vi "Find Path.vi"(7 "Map Colour Coding":T1={"Empty"=16448250, "Walls"=0, "Path"=3381759, "Waypoint"=16860, "Goal"=16711680}, 8 "Diagonals":bool, 9 "Ball Data":T3, 10 "Goal":cluster{"X":sgl, "Y":sgl}, 11 "Maze Walls":T2) -> (1 "Waypoints":i32[][](array[numeric]), 2 "Full Path":i32[][](array[numeric]), 3 "Image Out":T2)   [LabVIEW 2012]
uses:
  <vilib>/vision/Image Controls.llb/IMAQ Image.ctl
  <vilib>/robotics/Navigation/shared/WorldMap/OccupancyGridWorldMap/NI_Robotics_OccupancyGridWorldMap.lvclass
  <vilib>/robotics/Navigation/NI_Robotics_Navigation .lvlib
  <vilib>/vision/NI_Vision_Development_Module.lvlib
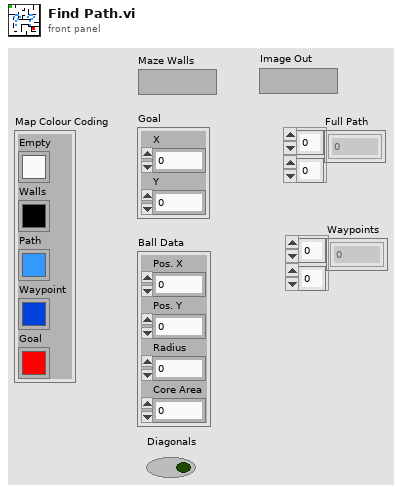
[diagram p1: front panel]
types:
  T1 = cluster{"Empty":u32, "Walls":u32, "Path":u32, "Waypoint":u32, "Goal":u32}
  T2 = typedef "IMAQ Image.ctl" = refnum<image>
  T3 = cluster{"Pos. X":i32, "Pos. Y":i32, "Radius":i32, "Core Area":i32}
  T4 = typedef "Image Type" = u32
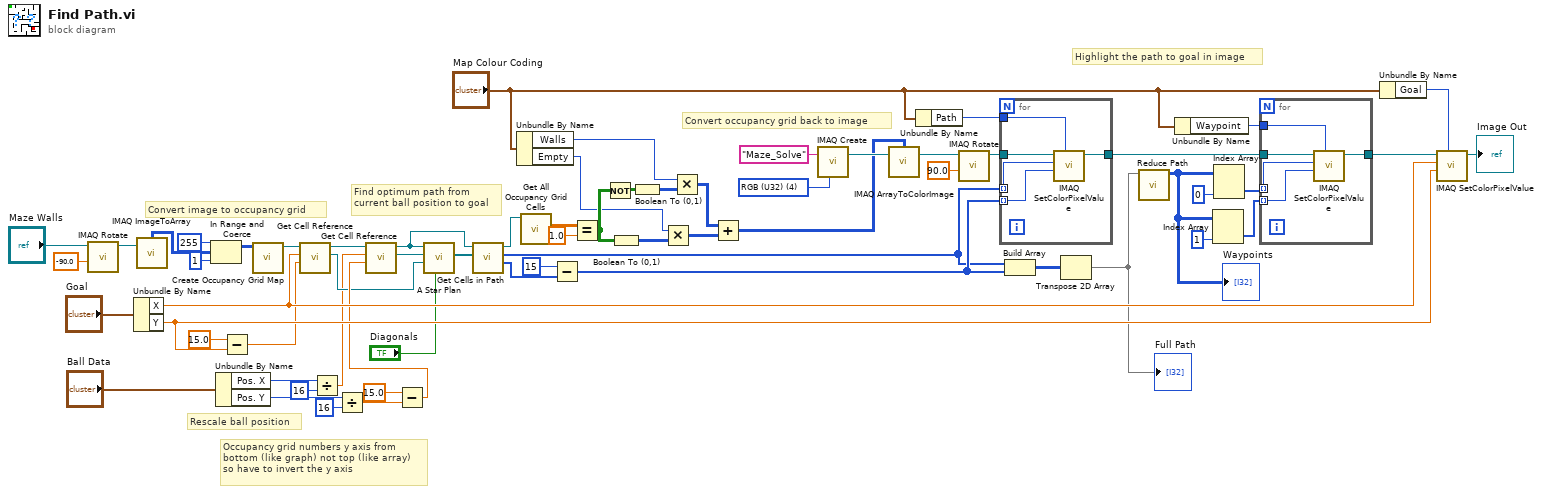
[diagram p0: block diagram]
diagram:
  w53 = T4 4 items=["Grayscale (U8)", "Grayscale (I16)", "Grayscale (SGL)", "Complex (CSG)", "RGB (U32)", "HSL (U32)", "RGB (U64)", "Grayscale (U16)"] ("Image Type")
  # "Highlight the path to goal in image"
  # "Convert occupancy grid back to image"
  # "Find optimum path from\ncurrent ball position to goal"
  # "Convert image to occupancy grid"
  # "Occupancy grid numbers y axis from\nbottom (like graph) not top (like array)\nso have to invert the y axis"
  # "Rescale ball position"
  n1 = call "IMAQ Rotate"("Angle (degrees)"=sgl -90.0, "Image Src"="Maze Walls") -> ("Image Dst Out"=w44:T2)  [unwired: 8 in, 1 out]
  n2 = Unbundle By Name("Goal") -> ("X"=w60:sgl, "Y"=w61:sgl)
  n3 = call "IMAQ ImageToArray"("Image"=w44) -> ("Image Pixels (U8)"=w25:u8[][])  [unwired: 3 in, 4 out]
  n4 = In Range and Coerce(upper limit=u8 255, x=w25, lower limit=u8 1) -> (coerced(x)=w24:u8[][])  [unwired: 1 out]
  n5 = Unbundle By Name("Ball Data") -> ("Pos. X"=w31:i32, "Pos. Y"=w34:i32)
  n6 = Subtract(x=sgl 15.0, y=w61) -> (x-y=w51:sgl)
  n7 = call <vilib>:"Create Occupancy Grid Map.vi"("occupancy grid"=w24) -> ("map reference out"=w42:refnum<data-value>)  [unwired: 9 in, 1 out]
  n8 = call <vilib>:"Get Cell Reference.vi"("y"=w51, "x"=w60, "map reference in"=w42) -> ("cell reference"=w39:refnum<data-value>, "map reference out"=w36:refnum<data-value>)  [unwired: 5 in, 2 out]
  n9 = Divide(x=w31, y=16) -> (x/y=w37:dbl)
  n10 = Divide(x=w34, y=16) -> (x/y=w48:dbl)
  n11 = Subtract(x=15.0, y=w48) -> (x-y=w49:dbl)
  n12 = call <vilib>:"Get Cell Reference.vi"("y"=w49, "x"=w37, "map reference in"=w36) -> ("cell reference"=w38:refnum<data-value>, "map reference out"=w41:refnum<data-value>)  [unwired: 5 in, 2 out]
  n13 = call <vilib>:"A Star Plan.vi"("Diagonals"="Diagonals", "goal reference"=w39, "start reference"=w38, "map reference in"=w41) -> ("path references"=w40:refnum<data-value>[])  [unwired: 4 in, 3 out]
  n14 = call <vilib>:"Get Cells in Path.vi"("path references"=w40, "map reference in"=w41) -> ("y coordinates"=w58:i32[], "x coordinates"=w62:i32[], "map reference out"=w46:refnum<data-value>)  [unwired: 6 in, 1 out]
  n15 = Unbundle By Name("Map Colour Coding") -> ("Walls"=w5:u32, "Empty"=w6:u32)
  n16 = call <vilib>:"Get All Occupancy Grid Cells.vi"("map reference in"=w46) -> ("occupancy grid"=w22:dbl[][])  [unwired: 8 in, 2 out]
  n17 = Subtract(x=15, y=w58) -> (x-y=w63:i32[])
  n18 = Equal?(x=w22, y=1.0) -> (x = y?=w13:bool[][])
  n19 = Not(x=w13) -> (.not. x?=w12:bool[][])
  n20 = Boolean To (0,1)(Boolean=w13) -> (0, 1=w7:i16[][])
  n21 = Boolean To (0,1)(Boolean=w12) -> (0, 1=w11:i16[][])
  n22 = Multiply(x=w6, y=w7) -> (x*y=w10:u32[][])
  n23 = Multiply(x=w5, y=w11) -> (x*y=w9:u32[][])
  n24 = Add(x=w9, y=w10) -> (x+y=w8:u32[][])
  n25 = call "IMAQ Create"("Image Name"="Maze_Solve", "Image Type"=w53) -> ("New Image"=w55:T2)  [unwired: 3 in, 1 out]
  n26 = call "IMAQ ArrayToColorImage"("Image Pixels (U32)"=w8, "Image"=w55) -> ("Image Out"=w56:T2)  [unwired: 3 in, 1 out]
  n27 = Unbundle By Name("Map Colour Coding") -> ("Path"=w4:u32)
  n28 = call "IMAQ Rotate"("Angle (degrees)"=sgl 90.0, "Image Src"=w56) -> ("Image Dst Out"=w59:T2)  [unwired: 8 in, 1 out]
  n29 = for {
    tunnel: w59 -> [w69]
    tunnel: w62 -> [w68] mode=indexing
    tunnel: w63 -> [w67] mode=indexing
    tunnel: [w66] -> w16
    tunnel: w4 -> [w65]
    n30 = call "IMAQ SetColorPixelValue"("Pixel Value (U32)"=w65, "Y Coordinate"=w67, "X Coordinate"=w68, "Image"=w69) -> ("Image Out"=w66:T2)  [unwired: 6 in, 1 out]
  }
  n31 = Build Array(w62, w63) -> (w64:i32[][])
  n32 = Transpose 2D Array(2D array=w64) -> (transposed array=w17:i32[][])
  "Full Path" <- w17
  n33 = call "Reduce Path.vi"("Path in"=w17) -> ("Reduced Path"=w14:i32[][])  [unwired: 10 in]
  "Waypoints" <- w14
  n34 = Unbundle By Name("Map Colour Coding") -> ("Waypoint"=w3:u32)
  n35 = Index Array(array=w14, index (col)=1 ("disabled index (col)")) -> (element=w18:i32[])  [unwired: 1 in]
  n36 = Index Array(array=w14, index (col)=0 ("disabled index (col)")) -> (element=w21:i32[])  [unwired: 1 in]
  n37 = for {
    tunnel: w16 -> [w74]
    tunnel: w21 -> [w73] mode=indexing
    tunnel: w18 -> [w72] mode=indexing
    tunnel: [w71] -> w15
    tunnel: w3 -> [w70]
    n38 = call "IMAQ SetColorPixelValue"("Pixel Value (U32)"=w70, "Y Coordinate"=w72, "X Coordinate"=w73, "Image"=w74) -> ("Image Out"=w71:T2)  [unwired: 6 in, 1 out]
  }
  n39 = Unbundle By Name("Map Colour Coding") -> ("Goal"=w1:u32)
  n40 = call "IMAQ SetColorPixelValue"("Pixel Value (U32)"=w1, "Y Coordinate"=w61, "X Coordinate"=w60, "Image"=w15) -> ("Image Out"=→"Image Out":T2)  [unwired: 6 in, 1 out]
